vi "open_output.vi"(10 "Output File Header":string, 11 "Output Folder Path":path) -> (1 "Output File Name":string, 2 "Output File Path":path, 3 "refnum out":refnum<file>)   [LabVIEW 2016]
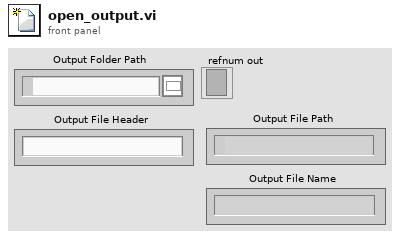
[diagram p1: front panel]
types:
  T1 = enum16{"open", "replace", "create", "open or create", "replace or create", "replace or create with confirmation"}
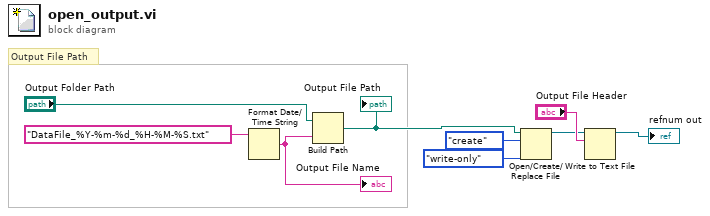
[diagram p0: block diagram]
diagram:
  # "Output File Path"
  n1 = Format Date/Time String(time format string (%c)="DataFile_%Y-%m-%d_%H-%M-%S.txt") -> (date/time string=w8:string)  [unwired: 2 in]
  "Output File Name" <- w8
  n2 = Build Path(base path="Output Folder Path", name or relative path=w8) -> (appended path=w4:path)
  "Output File Path" <- w4
  n3 = Open/Create/Replace File(file path (use dialog)=w4, operation (0:open)=T1."create", access (0:read/write)=enum16{"read/write", "read-only", "write-only"}."write-only") -> (refnum out=w2:refnum<file>)  [unwired: 3 in, 2 out]
  n4 = Write to Text File(file (use dialog)=w2, text="Output File Header") -> (refnum out=→"refnum out":refnum<file>)  [unwired: 2 in, 2 out]
